vi "CheckRef.vi"(8 "error in (no error)":errorcluster, 11 "Progress Bar":refnum<data-value>) -> (0 "error out":errorcluster, 3 "Progress Bar":refnum<data-value>)   [LabVIEW 2020, in "Progress Bar.lvclass"]
doc: "Checks to see if the ref is valid. If it's not, then create a valid ref (and store it for subsequent calls)\n\nCopyright: MGI\nAuthored by: Derek Trepanier"
uses:
  <userlib>/_MGI/User Interface/Progress Bar/Progress Bar.lvclass
  <userlib>/_MGI/User Interface/Progress Bar/Progress Bar.lvclass/Progress Bar.ctl
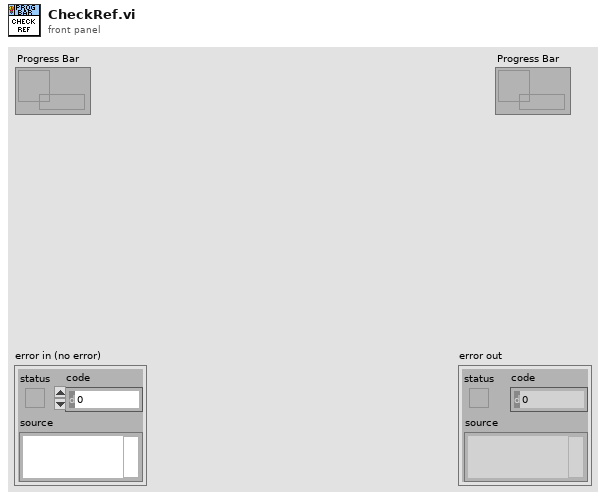
[diagram p1: front panel]
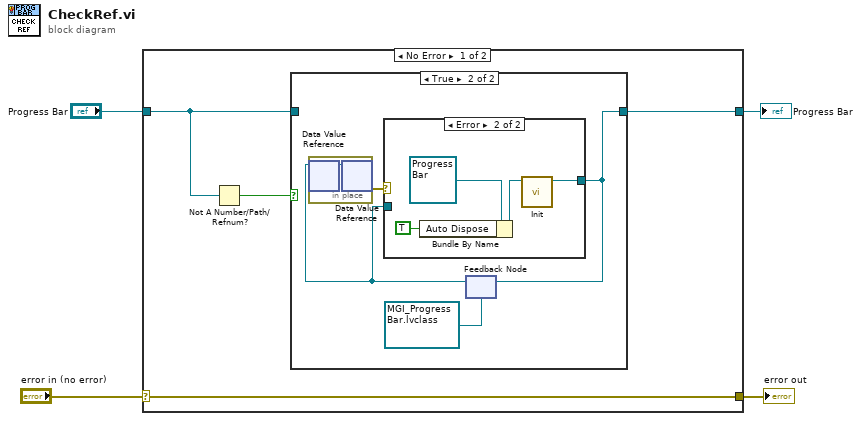
[diagram p0: block diagram]
diagram:
  n1 = case shown="No Error" "error in (no error)" {
    selector: "error in (no error)" -> [w8 w21]
    tunnel: [w8 w21] -> w3
    tunnel: [w5 w20] -> w2
    tunnel: "Progress Bar" -> [w6 w20]
    frame No Error {
      n2 = Not A Number/Path/Refnum?(number/path/refnum=w6) -> (NaN/Path/Refnum?=w7:bool)
      n3 = case shown="True" w7 {
        tunnel: [w9 w13] -> w5
        tunnel: w6 -> [w9 _]
        frame False {
        }
        frame True {
          n4 = feedback #1(refnum<data-value> refnum ("data value reference")) -> (w11:refnum<data-value>)
          n5 = in-place {
            n6 = in-place-dvr #2(w11) -> (w14:refnum<class "Progress Bar.lvclass">)  [unwired: 1 out]
            n7 = in-place-dvr #2(w14) -> (w10:errorcluster)  [unwired: 1 out]
          }
          n8 = case shown="Error" w10 {
            tunnel: [w15 w19] -> w13
            tunnel: w11 -> [w15 _]
            frame No Error {
            }
            frame Error {
              n9 = Bundle By Name(cluster=refnum<class "Progress Bar.lvclass"> refnum ("MGI_Progress Bar in"), "Auto Dispose"=TRUE) -> (w17:refnum<class "Progress Bar.lvclass">)
              n10 = call <userlib>:"Init.vi"("MGI_Progress Bar in"=w17) -> ("Progress Bar"=w19:refnum<data-value>)  [unwired: 9 in, 1 out]
            }
          }
          n11 = feedback-in #1(w13) -> ()
        }
      }
    }
    frame Error {
    }
  }
  "error out" <- w3
  "Progress Bar" <- w2
